vi "Find Balls.vi"(7 "Color Components":T3={"Hue"={110.0, 142.0}, "Sat"={138.0, 255.0}, "Val"={139.0, 198.0}} {"Val" scale=0.0..255.0; "Sat" scale=0.0..255.0; "Hue" scale=0.0..255.0 scale format="%#_3g"}, 9 "Score Cutoff":dbl(slide)=70.58823529411765 scale=0.0..100.0, 10 "Image Dst.":T1, 11 "Image Src.":T1) -> (0 "Ranked Objects":T2(array[cluster]) {"Score" format="%#.1g"}, 1 "MaskedImage":T1(plugin-control), 2 "Annotated Image":T1, 3 "Initial Image":T1)   [LabVIEW 2015]
uses:
  <vilib>/vision/Image Controls.llb/IMAQ Image.ctl
panel:
  in  "Targets":i32=3
  in  "Area Cutoff %":dbl=0.4
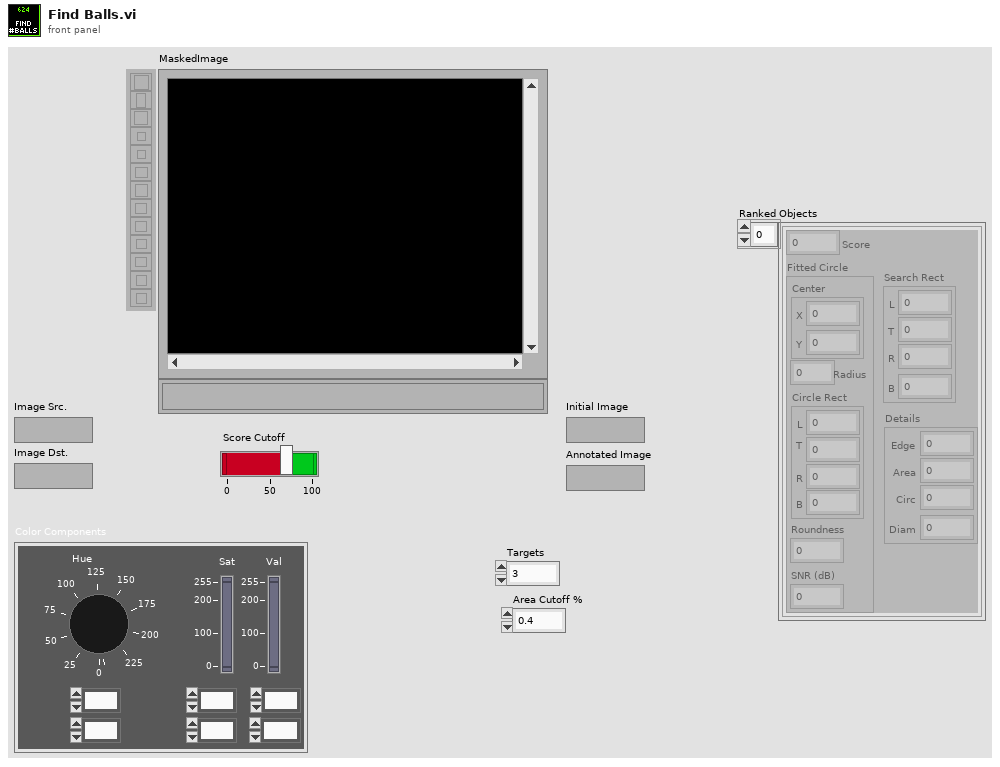
[diagram p1: front panel]
types:
  T1 = typedef "IMAQ Image.ctl" = refnum<image>
  T2 = cluster{"Score":sgl, "Fitted Circle":cluster{"Center":cluster{"X":sgl, "Y":sgl}, "Radius":dbl, "Circle Rect":cluster{"L":sgl, "T":sgl, "R":sgl, "B":sgl}, "Roundness":dbl, "SNR (dB)":dbl}, "Search Rect":cluster{"L":sgl, "T":sgl, "R":sgl, "B":sgl}, "Details":cluster{"Edge":sgl, "Area":sgl, "Circ":sgl, "Diam":sgl}}[]
  T3 = cluster{"Hue":cluster{dbl, dbl}, "Sat":cluster{dbl, dbl}, "Val":cluster{dbl, dbl}}
  T4 = cluster{"Circle Found":bool, "Fitted Circle":cluster{"Center":cluster{"X":sgl, "Y":sgl}, "Radius":dbl, "Center":cluster{"X":sgl, "Y":sgl}, "Radius":dbl, "Roundness":dbl, "Strength":dbl, "SNR (dB)":dbl}, "Array":dbl[], "Sorted Data":dbl[][]}[]
  T5 = cluster{"Score":dbl, "Fitted Circle":cluster{"Center (Pixels)":cluster{"X":sgl, "Y":sgl}, "Radius (Pixels)":dbl, "Circle Rect":cluster{"Left":sgl, "Top":sgl, "Right":sgl, "Bottom":sgl}, "Roundness (RW)":dbl, "Average SNR (dB)":dbl}, "Search Rect":cluster{"Left":sgl, "Top":sgl, "Right":sgl, "Bottom":sgl}, "Details":cluster{"Edges":sgl, "Circ/Rect":sgl, "Diam/Diam":sgl, "Circularity":sgl}}[]
  T6 = cluster{"Center (Pixels)":cluster{"X":sgl, "Y":sgl}, "Radius (Pixels)":dbl, "Circle Rect":cluster{"Left":sgl, "Top":sgl, "Right":sgl, "Bottom":sgl}, "Roundness (RW)":dbl, "Average SNR (dB)":dbl}
  T7 = cluster{"Left":sgl, "Top":sgl, "Right":sgl, "Bottom":sgl}
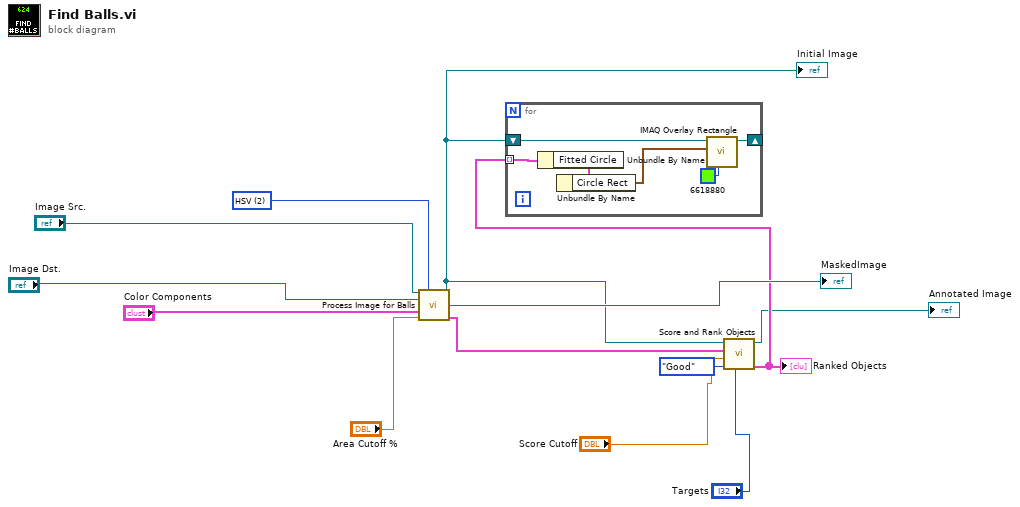
[diagram p0: block diagram]
diagram:
  w10 = u16 2 items=["RGB", "HSL", "HSV", "HSI"] ("Color Mode")
  n1 = call "Process Image for Balls.vi"("Src Image"="Image Src.", "Color Mode 2"=w10, "Image Dst"="Image Dst.", "Color"="Color Components", "Area Cutoff %"="Area Cutoff %") -> ("Src Image Out"=w5:T1, "First Threshold"=→"MaskedImage":T1, "Potential"=w4:T4)  [unwired: 7 in, 1 out]
  "Initial Image" <- w5
  n2 = call "Score and Rank Objects.vi"("Targets"="Targets", "Annotations"=enum16{"None", "Good", "All"}."Good", "Score Limit"="Score Cutoff", "Object Info"=w4, "Image in"=w5) -> ("Object Info"=w3:T5, "Annotated Image"=→"Annotated Image":T1)  [unwired: 5 in]
  "Ranked Objects" <- w3
  n3 = for {
    shift-right: [w18] -> _
    shift-left: w5 -> [w19]
    tunnel: w3 -> [w17] mode=indexing
    n4 = Unbundle By Name(w17) -> ("Fitted Circle"=w15:T6)
    n5 = Unbundle By Name(w15) -> ("Circle Rect"=w14:T7)
    n6 = call "IMAQ Overlay Rectangle"("Color"=u32 6618880, "Rectangle"=w14, "Image"=w19) -> ("Image Out"=w18:T1)  [unwired: 7 in, 1 out]
  }
